vi "sql viewer.vi"(10 "SQL2":string, 11 "SQL1":string) -> ()   [LabVIEW 2014]
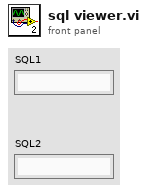
[diagram p1: front panel]
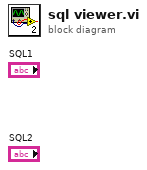
[diagram p0: block diagram]
diagram:
